vi "Write Index.vi"(8 "error in (no error)":errorcluster, 10 "Index":u16, 11 "NT Enum in":refnum<class "NT Enum.lvclass">) -> (0 "error out":errorcluster, 3 "NT Enum out":refnum<class "NT Enum.lvclass">)   [LabVIEW 2020, in "PV Access.lvlib" / "PV Data.lvlib" / "NT Enum.lvclass"]
uses:
  NT Enum.lvclass
  NT Enum.lvclass/NT Enum.ctl
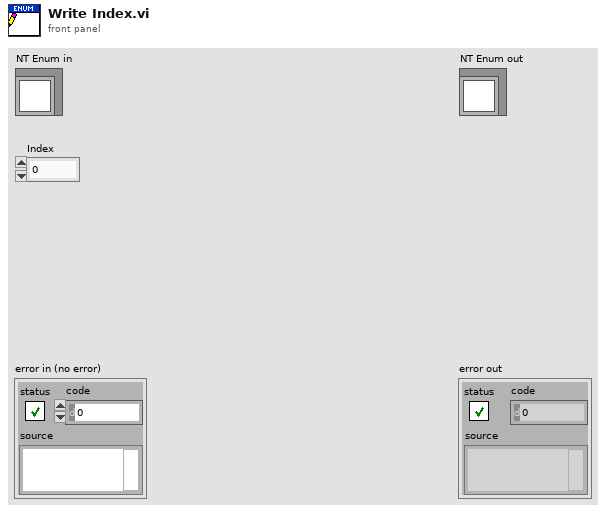
[diagram p1: front panel]
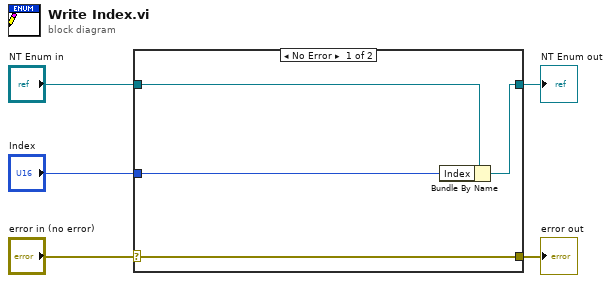
[diagram p0: block diagram]
diagram:
  n1 = case shown="No Error" "error in (no error)" {
    selector: "error in (no error)" -> [w9 w10]
    tunnel: [w9 w10] -> w4
    tunnel: [w7 w11] -> w2
    tunnel: "NT Enum in" -> [w8 w11]
    tunnel: "Index" -> [w6 _]
    frame No Error {
      n2 = Bundle By Name(cluster=w8, "Index"=w6) -> (w7:refnum<class "NT Enum.lvclass">)
    }
    frame Error {
    }
  }
  "error out" <- w4
  "NT Enum out" <- w2
